vi "test_Create Global MetaData Channel_error on empty name.vi"(8 "error in (no error)":errorcluster, 11 "TestCase in":refnum<class "Instrument Addon Scripting API Channels Unit Tests.lvclass">) -> (0 "error out":errorcluster, 3 "TestCase out":refnum<class "Instrument Addon Scripting API Channels Unit Tests.lvclass">)   [LabVIEW 2019, in "Instrument Addon Scripting API Channels Unit Tests.lvclass"]
uses:
  Instrument Addon Scripting API Channels Unit Tests.lvclass
  <vilib>/addons/_JKI Toolkits/VI Tester/TestCase.llb/TestCase.lvclass
  APIs/Scripting API/Instrument Addon Scripting API.lvlib
  APIs/Scripting API/TypeDefs/Array Element.ctl
  Addon/Addon Shared/Types/Type Cast Type.ctl
  Addon/Addon Shared/Instrument Addon Shared.lvlib
  Addon/Addon Shared/Types/Endian.ctl
  APIs/Scripting API/TypeDefs/Array Type Cast Settings.ctl
  APIs/Scripting API/Channels/Create Global MetaData Channel - Array - Type Cast.vi
  C:/Program Files (x86)/National Instruments/LabVIEW 2019/vi.lib/addons/_JKI Toolkits/VI Tester/TestCase.llb/TestCase.lvclass
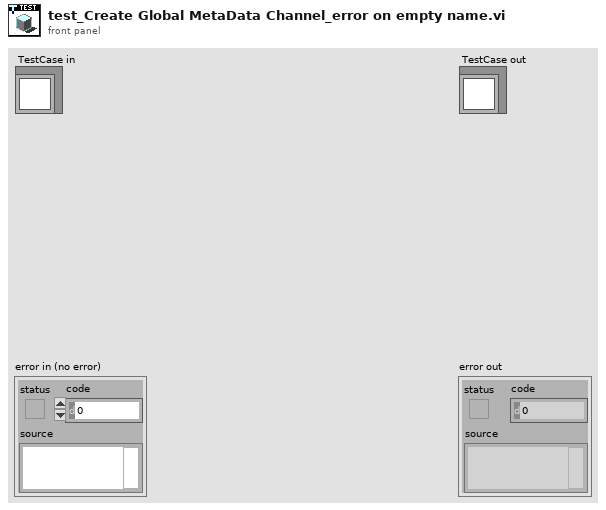
[diagram p1: front panel]
types:
  T1 = typedef "Instrument Addon Scripting API.lvlib/Array Type Cast Settings.ctl" = cluster{"Elements":T2[], "Delimiter":string, "Type":T3, "Endian":T4}
  T2 = typedef "Instrument Addon Scripting API.lvlib/Array Element.ctl" = cluster{"Name":string, "Default Value":dbl, "Units":string}
  T3 = typedef "Instrument Addon Shared.lvlib/Type Cast Type.ctl" = enum16{"DBL", "SGL", "U64", "U32", "U16", "U8", "I64", "I32", "I16", "I8"}
  T4 = typedef "Instrument Addon Shared.lvlib/Endian.ctl" = enum16{"Native", "Little", "Big"}
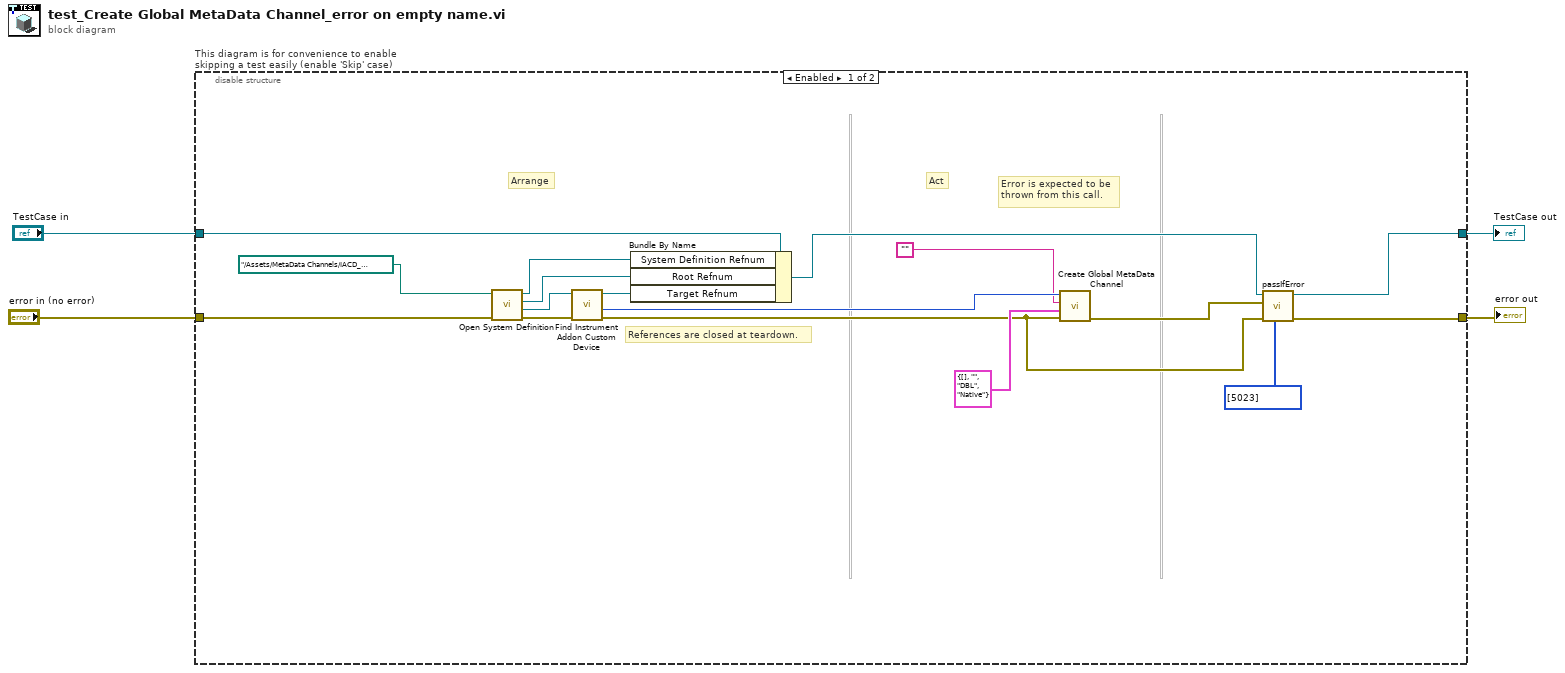
[diagram p0: block diagram]
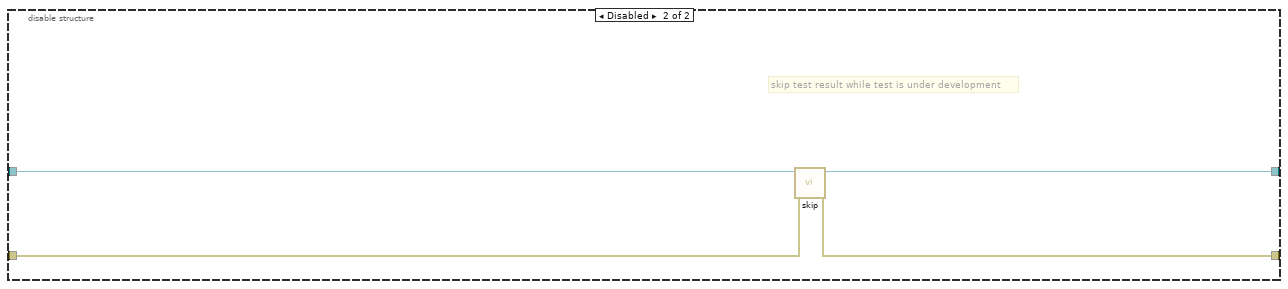
[diagram p2: hidden frame]
diagram:
  n1 = disable-structure "This diagram is for convenience to enable skipping a test easily (enable 'Skip' case)" shown="Enabled" {
    disable-tunnel: "TestCase in" -> [w15 w25]
    disable-tunnel: [w14 w23] -> w1
    disable-tunnel: [w13 w24] -> w3
    disable-tunnel: "error in (no error)" -> [w21 w22]
    frame Enabled {
      # "Error is expected to be\nthrown from this call."
      # "References are closed at teardown."
      # "Act"
      # "Arrange"
      n2 = call "Open System Definition.vi"("error in (no error)"=w21, "System Definition File"=path "../Assets/MetaData Channels/IACD_channels.nivssdf") -> ("error out"=w19:errorcluster, "Target Refnum"=w20:refnum<k24>, "Root Refnum"=w17:refnum<k24>, "System Definition Refnum"=w16:refnum<k24>)  [unwired: 6 in]
      n3 = call "Find Instrument Addon Custom Device.vi"("error in"=w19, "target in"=w20) -> ("error out"=w8:errorcluster, "NodeID"=w7:u64, "target out"=w18:refnum<k24>)  [unwired: 7 in]
      n4 = Bundle By Name(cluster=w15, "System Definition Refnum"=w16, "Root Refnum"=w17, "Target Refnum"=w18) -> (w11:refnum<class "Instrument Addon Scripting API Channels Unit Tests.lvclass">)
      n5 = call-poly "Create Global MetaData Channel.vi"("error in (no error)"=w8, "settings"=T1 {"Elements"=[], "Delimiter"="", "Type"=enum."DBL", "Endian"=enum."Native"} ("Settings"), "channel name"="", "instrument addon refnum in"=w7) -> ("error out"=w9:errorcluster)  [unwired: 4 in, 3 out]
      n6 = call-dynamic "passIfError.vi"("passing error codes (default = any error code)"=i32[] [5023], "error in (no error)"=w8, "error"=w9, "TestCase in"=w11) -> ("error out"=w13:errorcluster, "TestCase out"=w14:refnum<class "Instrument Addon Scripting API Channels Unit Tests.lvclass">)  [unwired: 6 in]
    }
    frame Disabled {
      # "skip test result while test is under development"
      n7 = call <vilib>:"skip.vi"("error in (no error)"=w22, "TestCase in"=w25) -> ("error out"=w24:errorcluster, "TestCase out"=w23:refnum<class "Instrument Addon Scripting API Channels Unit Tests.lvclass">)  [unwired: 8 in]
    }
  }
  "error out" <- w3
  "TestCase out" <- w1
